vi "Close.vi"(8 "error in (no error)":errorcluster, 11 "NI-Sync in":refnum<class "NI-Sync.lvclass">) -> (0 "error out":errorcluster, 3 "NI-Sync out":refnum<class "NI-Sync.lvclass">)   [LabVIEW 2025, in "Synchronization.lvlib" / "NI-Sync.lvclass"]
uses:
  NI-Sync.lvclass
  NI-Sync.lvclass/NI-Sync.ctl
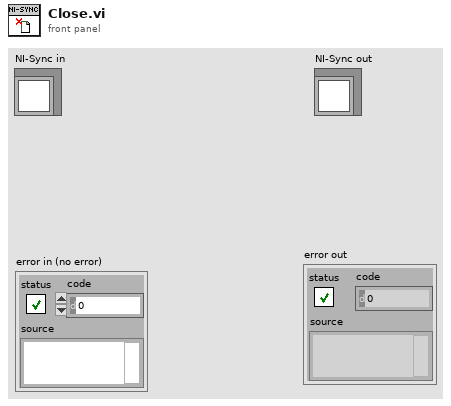
[diagram p1: front panel]
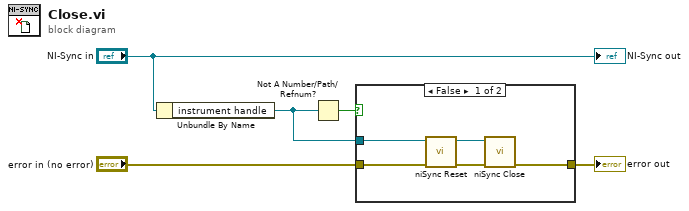
[diagram p0: block diagram]
diagram:
  n1 = Unbundle By Name("NI-Sync in") -> ("instrument handle"=w1:refnum<k15>)
  n2 = Not A Number/Path/Refnum?(number/path/refnum=w1) -> (NaN/Path/Refnum?=w2:bool)
  n3 = case shown="False" w2 {
    tunnel: "error in (no error)" -> [w8 w11]
    tunnel: [w7 w11] -> w3
    tunnel: w1 -> [w6 _]
    frame False {
      n4 = call <instrlib>:"niSync Reset.vi"("error in (no error)"=w8, "instrument handle"=w6) -> ("error out"=w9:errorcluster, "instrument handle out"=w10:refnum<k15>)  [unwired: 8 in]
      n5 = call <instrlib>:"niSync Close.vi"("error in (no error)"=w9, "instrument handle"=w10) -> ("error out"=w7:errorcluster)  [unwired: 9 in]
    }
    frame True {
    }
  }
  "error out" <- w3
  "NI-Sync out" <- "NI-Sync in"
